vi "Read Pressure (mbar).vi"(8 "error in (no error)":errorcluster, 11 "LPS Barometric Pressure Sensor in":refnum<class "LPS Barometric Pressure Sensor.lvclass">) -> (0 "error out":errorcluster, 2 "Pressure (mbar/hPa)":dbl, 3 "LPS Barometric Pressure Sensor out":refnum<class "LPS Barometric Pressure Sensor.lvclass">)   [LabVIEW 2020, in "LPS Barometric Pressure Sensor.lvclass"]
uses:
  LPS Barometric Pressure Sensor.lvclass
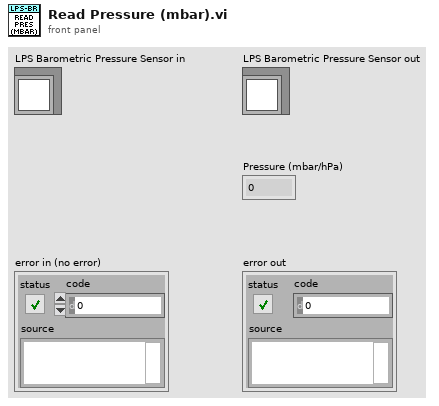
[diagram p1: front panel]
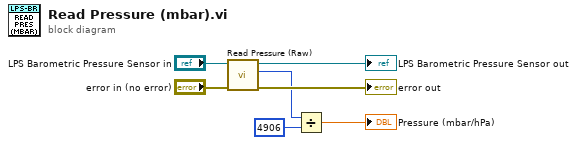
[diagram p0: block diagram]
diagram:
  n1 = call-dynamic "Read Pressure (Raw).vi"("error in (no error)"="error in (no error)", "LPS Barometer in"="LPS Barometric Pressure Sensor in") -> ("error out"=→"error out":errorcluster, "Raw Pressure"=w3:u32, "LPS Barometer out"=→"LPS Barometric Pressure Sensor out":refnum<class "LPS Barometric Pressure Sensor.lvclass">)  [unwired: 7 in]
  n2 = Divide(x=w3, y=i16 4906) -> (x/y=→"Pressure (mbar/hPa)":dbl)
